vi "Run Bfr Rx - CachedSize - Add to Cache.vi"(5 "Data Size in":u64, 7 "Data in":u8[](array[numeric]), 8 "error in (no error)":errorcluster, 11 "Cached Buffer in":T1 {"Cache Buffer" format="%016x"}) -> (0 "error out":errorcluster, 3 "Cached Buffer out":T1 {"Cache Buffer" format="%016x"})   [LabVIEW 2016, in "UDP-Custom-Device Engine.lvlib"]
uses:
  UDP-Custom-Device Engine.lvlib
  Types/Engine - Buffered Rx Cached Buffer.ctl
  <vilib>/NI Veristand/VeriStand Data/Pointer Operations/Pointer.Read (U16).vi
  <vilib>/NI Veristand/VeriStand Data/Pointer Operations/Pointer.Write (U16).vi
  <vilib>/NI Veristand/VeriStand Data/Pointer Operations/Pointer.Write (I32).vi
  <vilib>/NI Veristand/VeriStand Data/Pointer Operations/Pointer.Write (1D U8).vi
  <vilib>/NI Veristand/VeriStand Data/Pointer Operations/Pointer.In-Place Read (U16).vi
  <vilib>/NI Veristand/VeriStand Data/VeriStand Data.lvlib
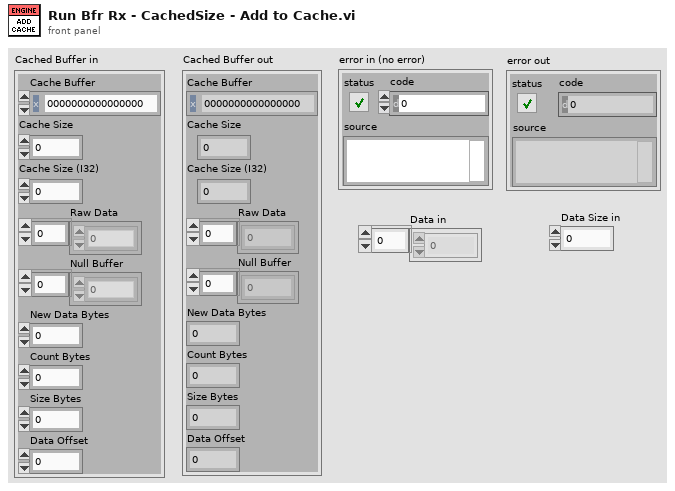
[diagram p1: front panel]
types:
  T1 = typedef "UDP-Custom-Device Engine.lvlib/Engine - Buffered Rx Cached Buffer.ctl" = cluster{"Cache Buffer":u64, "Cache Size":u64, "Cache Size (I32)":i32, "Raw Data":u8[], "Null Buffer":u8[], "New Data Bytes":u64, "Count Bytes":u64, "Size Bytes":u64, "Data Offset":u64}
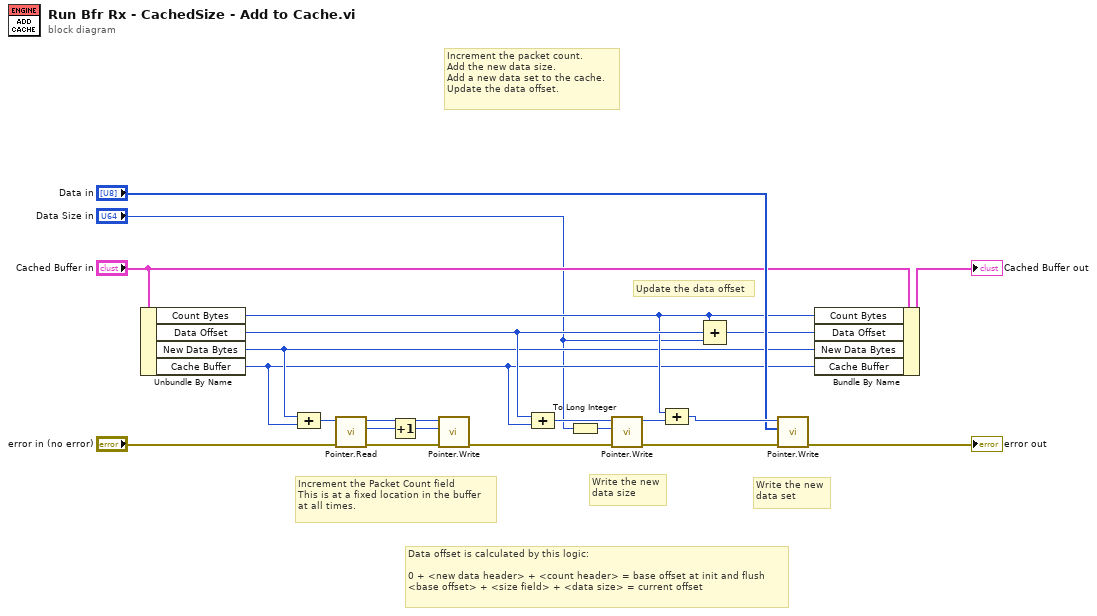
[diagram p0: block diagram]
diagram:
  # "Data offset is calculated by this logic:\n\n0 + <new data header> + <count header> = base offset at init and flush\n<base offset> + <size field> + <data size> = current offset"
  # "Update the data offset"
  # "Write the new\ndata set"
  # "Write the new\ndata size"
  # "Increment the Packet Count field\nThis is at a fixed location in the buffer\nat all times."
  # "Increment the packet count.\nAdd the new data size.\nAdd a new data set to the cache.\nUpdate the data offset."
  n1 = Unbundle By Name("Cached Buffer in") -> ("Count Bytes"=w4:u64, "Data Offset"=w9:u64, "New Data Bytes"=w3:u64, "Cache Buffer"=w2:u64)
  n2 = Compound Arithmetic op=ADD(w3, w2) -> (w22:u64)
  n3 = call-poly <vilib>:"Pointer.Read.vi"("error in (no error)"="error in (no error)", "pointer in"=w22) -> ("error out"=w20:errorcluster, "value"=w18:u16, "pointer out"=w19:u64)  [unwired: 7 in]
  n4 = Increment(x=w18) -> (x+1=w17:u16)
  n5 = call-poly <vilib>:"Pointer.Write.vi"("error in (no error)"=w20, "value"=w17, "pointer in"=w19) -> ("error out"=w15:errorcluster)  [unwired: 6 in, 2 out]
  n6 = Compound Arithmetic op=ADD(w9, w2) -> (w16:u64)
  n7 = To Long Integer(number="Data Size in") -> (32bit integer=w14:i32)
  n8 = call-poly <vilib>:"Pointer.Write.vi"("error in (no error)"=w15, "value"=w14, "pointer in"=w16) -> ("error out"=w13:errorcluster, "pointer out"=w11:u64)  [unwired: 6 in, 1 out]
  n9 = Compound Arithmetic op=ADD(w4, w11) -> (w10:u64)
  n10 = Compound Arithmetic op=ADD(w4, w9, "Data Size in") -> (w5:u64)
  n11 = call-poly <vilib>:"Pointer.Write.vi"("error in (no error)"=w13, "values"="Data in", "pointer in"=w10) -> ("error out"=→"error out":errorcluster)  [unwired: 6 in, 2 out]
  n12 = Bundle By Name(cluster="Cached Buffer in", "Count Bytes"=w4, "Data Offset"=w5, "New Data Bytes"=w3, "Cache Buffer"=w2) -> (→"Cached Buffer out":T1)
